vi "Main.vi"() -> ()   [LabVIEW 2020]
doc: "Use this template to build a simple state machine design pattern. Each state executes code and determines which state to transition to."
uses:
  controls/State.ctl
  controls/Data.ctl
  DAQmx_settings.ctl
  <vilib>/DAQmx/create/channels.llb/DAQmx Create Channel (AI-Voltage-Basic).vi
  <vilib>/DAQmx/configure/timing.llb/DAQmx Timing (Sample Clock).vi
  <vilib>/daqmxs/DAQmx Read sim (Analog Wfm 1Chan NSamp).vi
  <vilib>/Waveform/WDTOps.llb/WDT Append Waveforms DBL.vi
  <vilib>/measure/mamon.llb/Waveform Peak Detection for 1 Chan.vi
  <vilib>/Utility/TDMS File Viewer/NI_TDMS File Viewer.lvlib
  <vilib>/daqmxs/DAQmx sim.lvlib
  <vilib>/measure/NI_MAPro.lvlib
panel:
  out "Waves found":i32
  out "Amplitudes":dbl[](array[numeric]) format="%.2p"
  out "Locations":dbl[](array[numeric]) format="%.2p"
  in  "threshold":dbl format="%.2p"
  out "Waveform Graph 2":waveform(dbl)(graph)
  in  "Save Button":bool
  out "Waveform Graph":waveform(dbl)(graph)
  in  "Stop 2":bool
  in  "Record Button":bool
  in  "Open Button":bool
  in  "physical channels":tag="Dev1/ai0"
  in  "Sample rate":dbl=1000.0 format="%0.2f"
  in  "samples per channel":dbl=100.0
  in  "minimum value":dbl=-5.0 format="%0.2f"
  in  "maximum value":dbl=8.0 format="%0.2f"
  in  "Exit":bool
  # "Settings"
  # "TDMS"
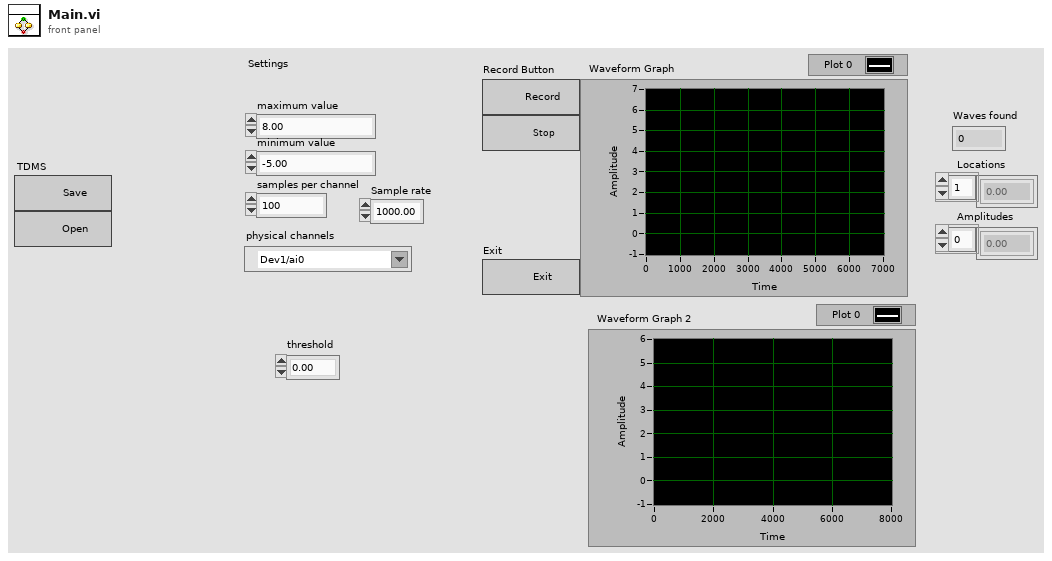
[diagram p1: front panel]
types:
  T1 = typedef "DAQmx_settings.ctl" = cluster{"maximum value":dbl, "minimum value":dbl, "samples per channel":dbl, "Sample rate":dbl, "physical channels":tag, "sample mode":i32, "Itterations":u16}
  T2 = typedef "Data.ctl" = cluster{"Stop sampling":bool, "Waveform":waveform(dbl), "task":refnum<k21>}
  T3 = typedef "State.ctl" = enum16{"Initialize", "Wait for Event", "TDMS save", "Start sampling", "Detect Wave", "Sampling", "Stop sampling", "Open file", "Exit"}
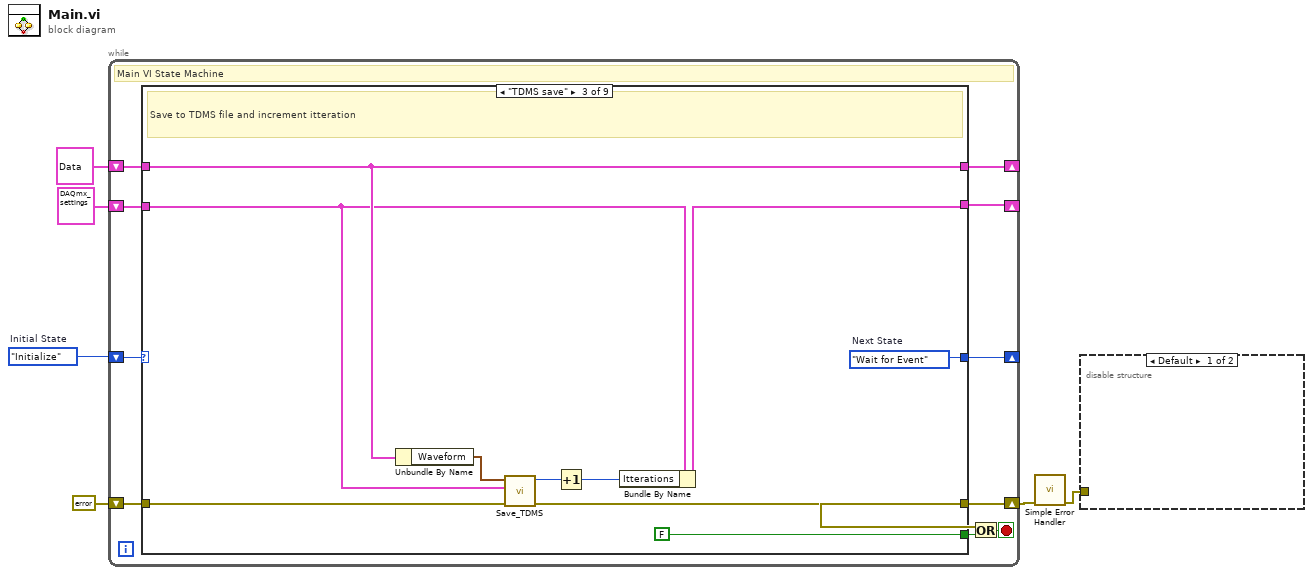
[diagram p0: block diagram]
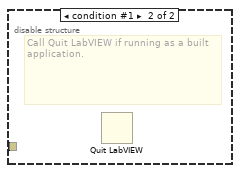
[diagram p2: hidden frame]
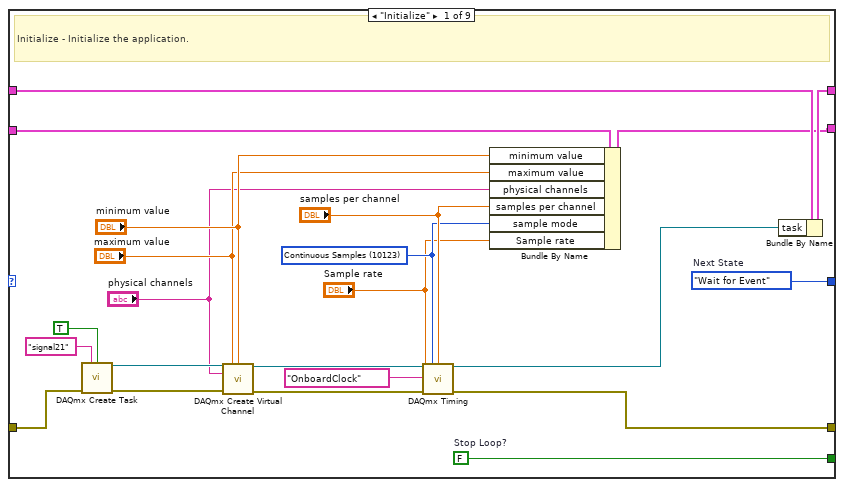
[diagram p3: hidden frame]
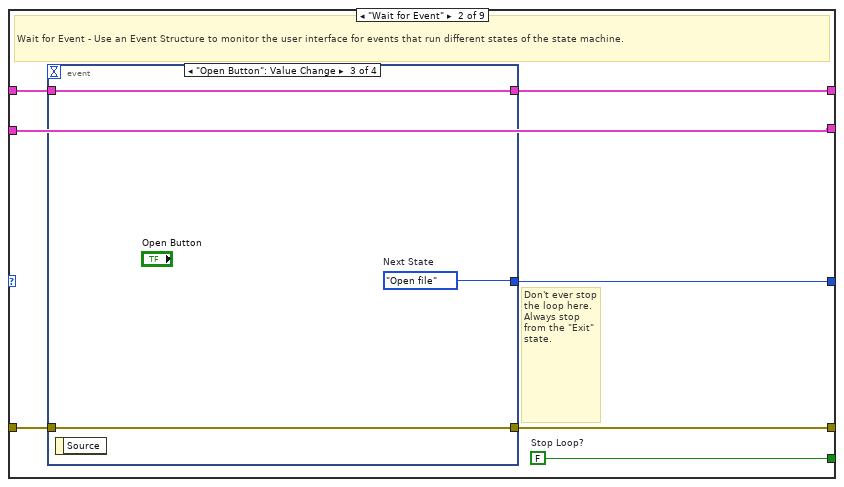
[diagram p4: hidden frame]
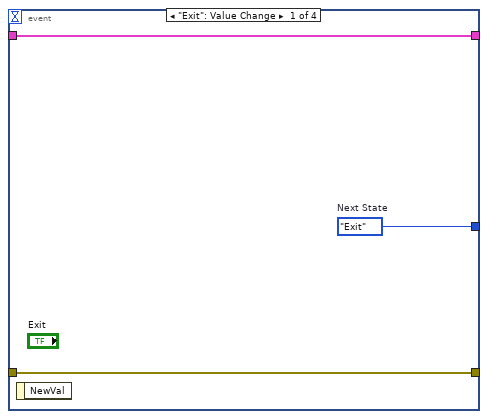
[diagram p5: hidden frame]
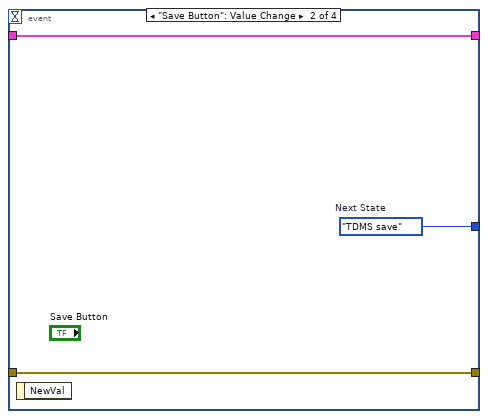
[diagram p6: hidden frame]
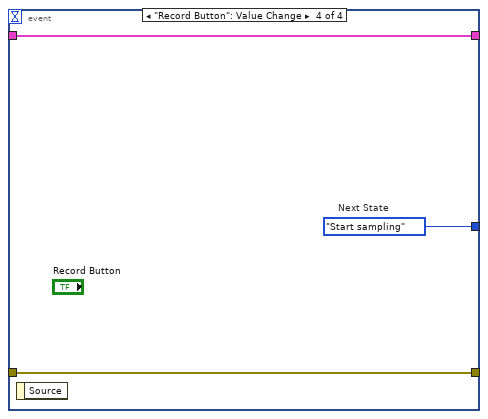
[diagram p7: hidden frame]
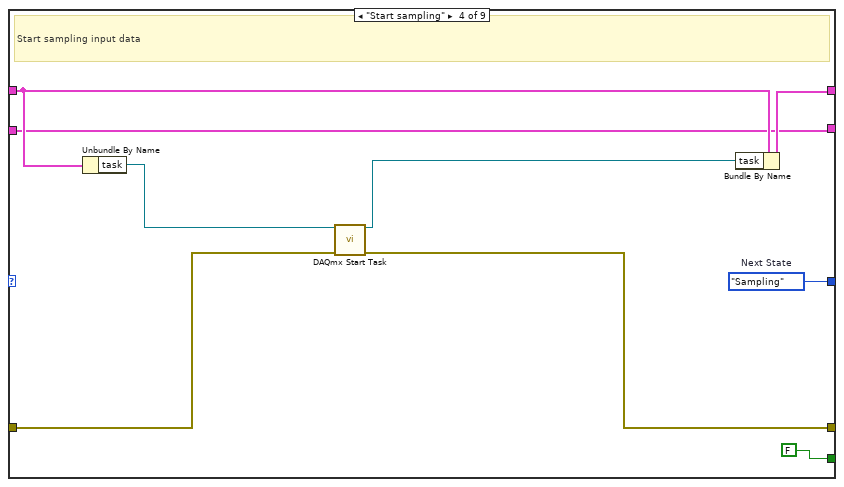
[diagram p8: hidden frame]
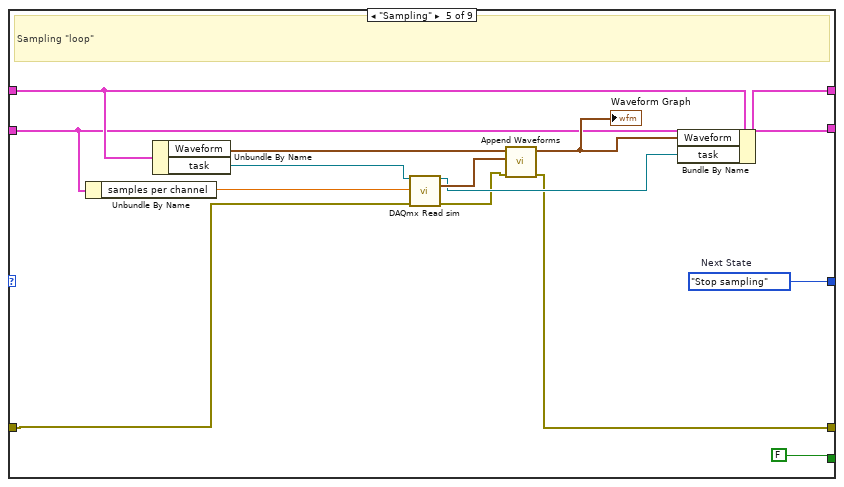
[diagram p9: hidden frame]
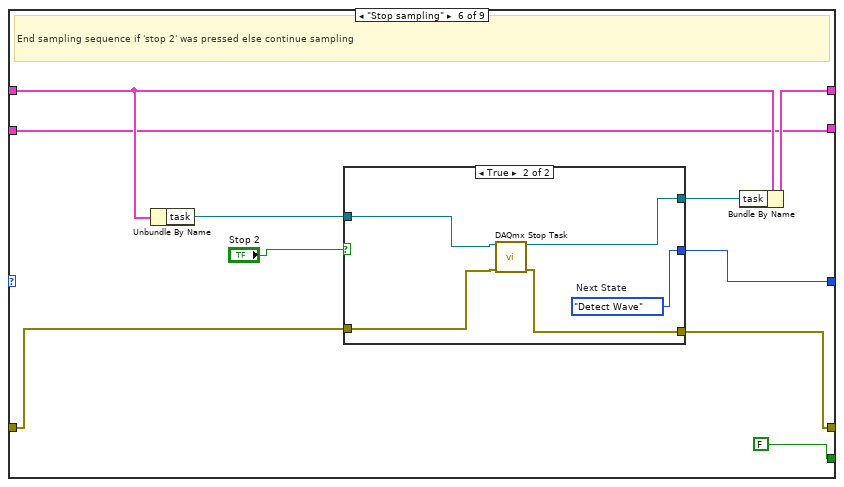
[diagram p10: hidden frame]
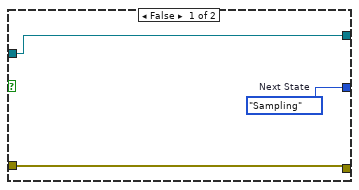
[diagram p11: hidden frame]
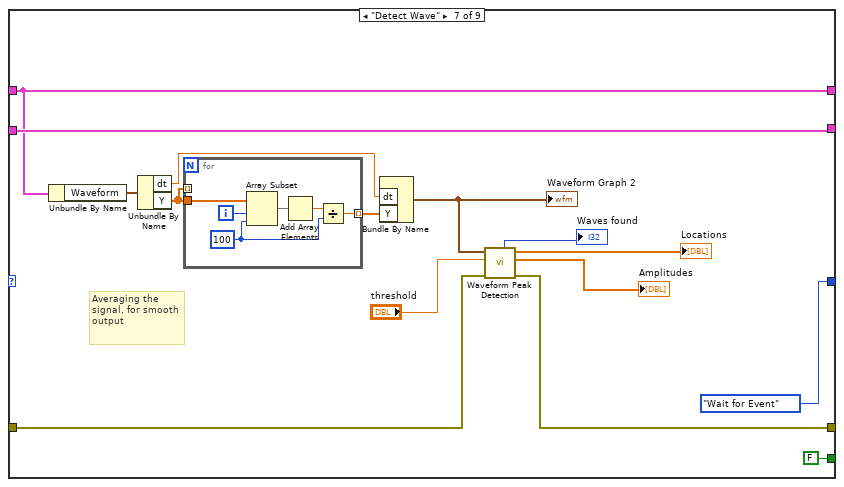
[diagram p12: hidden frame]
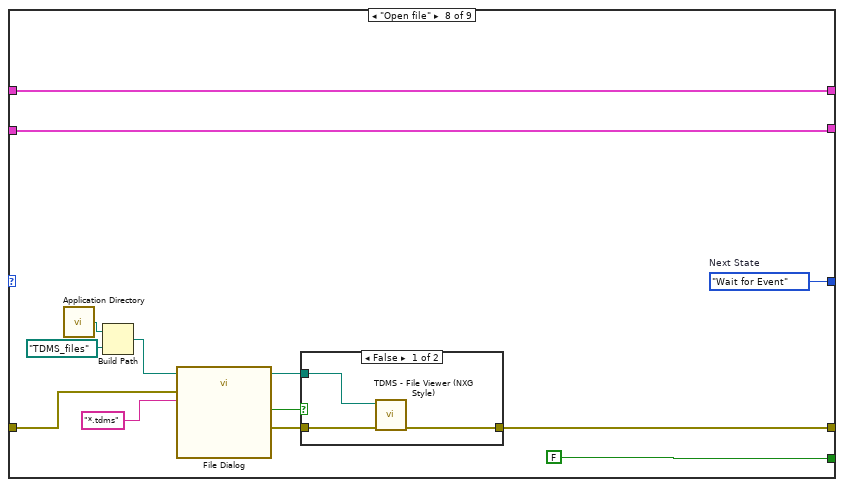
[diagram p13: hidden frame]
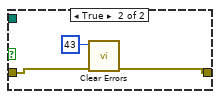
[diagram p14: hidden frame]
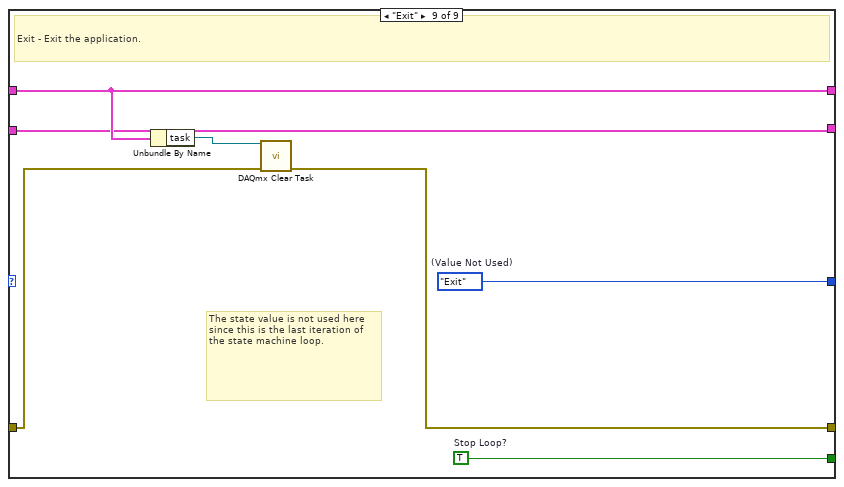
[diagram p15: hidden frame]
diagram:
  w6 = State."Initialize"  # Initial State
  n1 = while {
    shift-right: [w15] -> _
    shift-left: w6 -> [w16]
    shift-right: [w13] -> _
    shift-left: T2 {"Stop sampling"=FALSE, "Waveform"={"t0"=timestamp(0 s since 1904-01-01), "dt"=1.0, "Y"=[]}, "task"=""} ("Data") -> [w14]
    shift-right: [w9] -> w3
    shift-left: errorcluster {"status"=FALSE, "code"=0, "source"=""} ("error constant") -> [w12]
    shift-right: [w7] -> _
    shift-left: T1 {"maximum value"=8.0, "minimum value"=-5.0, "samples per channel"=100.0, "Sample rate"=1000.0, "physical channels"="Dev1/ai0", "sample mode"=10123, "Itterations"=0} -> [w8]
    stop <- w10 stop-if-true
    # "Main VI State Machine"
    n2 = case shown="\"TDMS save\"" w16 {
      tunnel: [w38 w45 w67 w75 w90 w99 State."Wait for Event" ("(Value Not Used)") w141 w155] -> w15
      tunnel: [w37 w44 FALSE ("Stop Loop?") FALSE FALSE FALSE FALSE ("Stop Loop?") FALSE w154] -> w11
      tunnel: w14 -> [w36 w43 w65 w74 w89 w100 w122 w142 w153]
      tunnel: [w35 w42 w65 w73 w88 w98 w122 w142 w153] -> w13
      tunnel: w12 -> [w32 w41 w64 w72 w81 w97 w113 w134 w151]
      tunnel: [w25 w40 w63 w71 w82 w96 w112 w139 w150] -> w9
      tunnel: w8 -> [w24 w39 w61 w68 w78 w91 w123 w130 w149]
      tunnel: [w23 w39 w60 w68 w78 w91 w123 w130 w149] -> w7
      frame "Initialize" {
        w18 = 10123 items=["Finite Samples"=10178, "Continuous Samples"=10123, "Hardware Timed Single Point"=12522] ("sample mode")
        w37 = FALSE  # Stop Loop?
        w38 = State."Wait for Event"  # Next State
        # "Initialize - Initialize the application."
        n3 = call <vilib>:"DAQmx Create Task.vi"("new task name"="signal21", "auto cleanup"=TRUE, "error in"=w32) -> ("task out"=w34:refnum<k21>, "error out"=w31:errorcluster)  [unwired: 11 in]
        n4 = call-poly <vilib>:"DAQmx Create Virtual Channel.vi"("task in"=w34, "maximum value"="maximum value", "minimum value"="minimum value", "physical channels"="physical channels", "error in"=w31) -> ("task out"=w33:refnum<k21>, "error out"=w30:errorcluster)  [unwired: 9 in]
        n5 = call-poly <vilib>:"DAQmx Timing.vi"("task/channels in"=w33, "sample mode"=w18, "samples per channel"="samples per channel", "rate"="Sample rate", "source"=tag "OnboardClock", "error in"=w30) -> ("task out"=w26:refnum<k21>, "error out"=w25:errorcluster)  [unwired: 8 in]
        n6 = Bundle By Name(cluster=w24, "minimum value"="minimum value", "maximum value"="maximum value", "physical channels"="physical channels", "samples per channel"="samples per channel", "sample mode"=w18, "Sample rate"="Sample rate") -> (w23:T1)
        n7 = Bundle By Name(cluster=w36, "task"=w26) -> (w35:T2)
      }
      frame "Wait for Event" {
        w44 = FALSE  # Stop Loop?
        # "Don't ever stop the loop here. Always stop from the \"Exit\" state."
        # "Wait for Event - Use an Event Structure to monitor the user interface for events that run different states of the state machine."
        n8 = event shown="[2] \"Open Button\": Value Change" {
          selector: _ -> [_ _ _ _]
          dyn-events: _ -> [_ _ _ _]
          timeout: _ -> [_ _ _ _]
          tunnel: [w48 w51 w52 w55] -> w45
          tunnel: w43 -> [w47 w49 w54 w57]
          tunnel: [w47 w49 w54 w57] -> w42
          tunnel: w41 -> [w46 w50 w53 w56]
          tunnel: [w46 w50 w53 w56] -> w40
          event "Exit": Value Change {
            w48 = State."Exit"  # Next State
            n9 = event-data() -> ()  [unwired: 1 in, 1 out]
          }
          event "Save Button": Value Change {
            w51 = State."TDMS save"  # Next State
            n10 = event-data() -> ()  [unwired: 1 in, 1 out]
          }
          event "Open Button": Value Change {
            w52 = State."Open file"  # Next State
            n11 = event-data() -> ()  [unwired: 1 in, 1 out]
          }
          event "Record Button": Value Change {
            w55 = State."Start sampling"  # Next State
            n12 = event-data() -> ()  [unwired: 1 in, 1 out]
          }
        }
      }
      frame "TDMS save" {
        w67 = State."Wait for Event"  # Next State
        # "Save to TDMS file and increment itteration"
        n13 = Unbundle By Name(w65) -> ("Waveform"=w62:waveform(dbl))
        n14 = call "Save_TDMS.vi"("error in (no error)"=w64, 10:w61, "Waveform"=w62) -> ("error out"=w63:errorcluster, "Numeric"=w59:u16)  [unwired: 7 in]
        n15 = Increment(x=w59) -> (x+1=w58:u16)
        n16 = Bundle By Name(cluster=w61, "Itterations"=w58) -> (w60:T1)
      }
      frame "Start sampling" {
        w75 = State."Sampling"  # Next State
        # "Start sampling input data"
        n17 = Unbundle By Name(w74) -> ("task"=w70:refnum<k21>)
        n18 = call <vilib>:"DAQmx Start Task.vi"("task/channels in"=w70, "error in"=w72) -> ("task out"=w69:refnum<k21>, "error out"=w71:errorcluster)  [unwired: 12 in]
        n19 = Bundle By Name(cluster=w74, "task"=w69) -> (w73:T2)
      }
      frame "Sampling" {
        w90 = State."Stop sampling"  # Next State
        # "Sampling \"loop\""
        n20 = Unbundle By Name(w78) -> ("samples per channel"=w77:dbl)
        n21 = Unbundle By Name(w89) -> ("Waveform"=w87:waveform(dbl), "task"=w84:refnum<k21>)
        n22 = call-poly <vilib>:"DAQmx Read sim.vi"("task/channels in"=w84, "number of samples per channel"=w77, "error in"=w81) -> ("task out"=w85:refnum<k21>, "data"=w86:waveform(dbl), "error out"=w83:errorcluster)  [unwired: 10 in]
        n23 = call-poly <vilib>:"Append Waveforms.vi"("error in (no error)"=w83, "waveform B"=w86, "waveform A"=w87) -> ("error out"=w82:errorcluster, "waveform out"=w79:waveform(dbl))  [unwired: 7 in]
        "Waveform Graph" <- w79
        n24 = Bundle By Name(cluster=w89, "Waveform"=w79, "task"=w85) -> (w88:T2)
      }
      frame "Stop sampling" {
        # "End sampling sequence if 'stop 2' was pressed else continue sampling"
        n25 = Unbundle By Name(w100) -> ("task"=w95:refnum<k21>)
        n26 = case shown="True" "Stop 2" {
          tunnel: [w103 w108] -> w99
          tunnel: w97 -> [w102 w107]
          tunnel: [w102 w106] -> w96
          tunnel: w95 -> [w101 w105]
          tunnel: [w101 w104] -> w94
          frame False {
            w103 = State."Sampling"  # Next State
          }
          frame True {
            w108 = State."Detect Wave"  # Next State
            n27 = call <vilib>:"DAQmx Stop Task.vi"("task/channels in"=w105, "error in"=w107) -> ("task out"=w104:refnum<k21>, "error out"=w106:errorcluster)  [unwired: 12 in]
          }
        }
        n28 = Bundle By Name(cluster=w100, "task"=w94) -> (w98:T2)
      }
      frame "Detect Wave" {
        # "Averaging the signal, for smooth output"
        n29 = Unbundle By Name(w122) -> ("Waveform"=w121:waveform(dbl))
        n30 = Unbundle By Name(w121) -> ("dt"=w116:dbl, "Y"=w118:dbl[])
        n31 = for {
          tunnel: w118 -> [_] mode=indexing
          tunnel: w118 -> [w128]
          tunnel: [w124] -> w117 mode=indexing
          i -> [w129]
          w125 = 100 ("length")
          n32 = Array Subset(array=w128, index=w129, length=w125) -> (w127:dbl[])
          n33 = Add Array Elements(numeric array=w127) -> (sum=w126:dbl)
          n34 = Divide(x=w126, y=w125) -> (x/y=w124:dbl)
        }
        n35 = Bundle By Name("dt"=w116, "Y"=w117) -> (w115:waveform(dbl))  [unwired: 1 in]
        "Waveform Graph 2" <- w115
        n36 = call-poly <vilib>:"Waveform Peak Detection.vi"("error in"=w113, "threshold"="threshold", "Signal In"=w115) -> ("error out"=w112:errorcluster, "Amplitudes"=→"Amplitudes":dbl[], "Locations"=→"Locations":dbl[], "# found"=→"Waves found":i32)  [unwired: 4 in, 1 out]
      }
      frame "Open file" {
        w141 = State."Wait for Event"  # Next State
        n37 = call <vilib>:"Application Directory.vi"() -> ("Application Directory"=w137:path)
        n38 = Build Path(base path=w137, name or relative path=path "TDMS_files") -> (appended path=w135:path)
        n39 = call "File Dialog"("start path"=w135, "error in"=w134, "pattern (all files)"="*.tdms") -> ("selected path"=w138:path, "cancelled"=w131:bool, "error out"=w133:errorcluster)  [unwired: 9 in, 1 out]
        n40 = case shown="False" w131 {
          tunnel: w133 -> [w145 w146]
          tunnel: [w144 w148] -> w139
          tunnel: w138 -> [w143 _]
          frame False {
            n41 = call <vilib>:"TDMS - File Viewer (NXG Style).vi"("error in"=w145, "file in"=w143) -> ("error out"=w144:errorcluster)  [unwired: 8 in, 1 out]
          }
          frame True {
            n42 = call <vilib>:"Clear Errors.vi"("error in (no error)"=w146, "specific error code to clear (0: all)"=43) -> ("error out"=w148:errorcluster)  [unwired: 4 in, 1 out]
          }
        }
      }
      frame "Exit" {
        w154 = TRUE  # Stop Loop?
        w155 = State."Exit"  # (Value Not Used)
        # "The state value is not used here since this is the last iteration of the state machine loop."
        # "Exit - Exit the application."
        n43 = Unbundle By Name(w153) -> ("task"=w152:refnum<k21>)
        n44 = call <vilib>:"DAQmx Clear Task.vi"("task in"=w152, "error in"=w151) -> ("error out"=w150:errorcluster)  [unwired: 13 in]
      }
    }
    n45 = Or(x=w9, y=w11) -> (x .or. y?=w10:bool)
  }
  n46 = call <vilib>:"Simple Error Handler.vi"("error in (no error)"=w3) -> ("error out"=w2:errorcluster)  [unwired: 4 in, 4 out]
  n47 = disable-structure shown="Default" {
    disable-tunnel: w2 -> [_ _]
    frame condition #0 (active) {
    }
    frame condition #1 {
      # "Call Quit LabVIEW if running as a built application."
      n48 = Quit LabVIEW() -> ()  [unwired: 1 in]
    }
  }
